vi "filtr2.vi"(8 "threshold":i32=1, 11 "input array":dbl[][](array[numeric])) -> (3 "output array":dbl[][](array[numeric]))   [LabVIEW 2015]
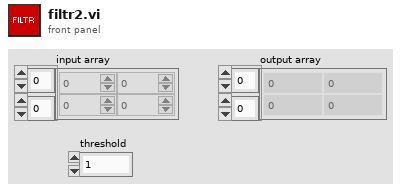
[diagram p1: front panel]
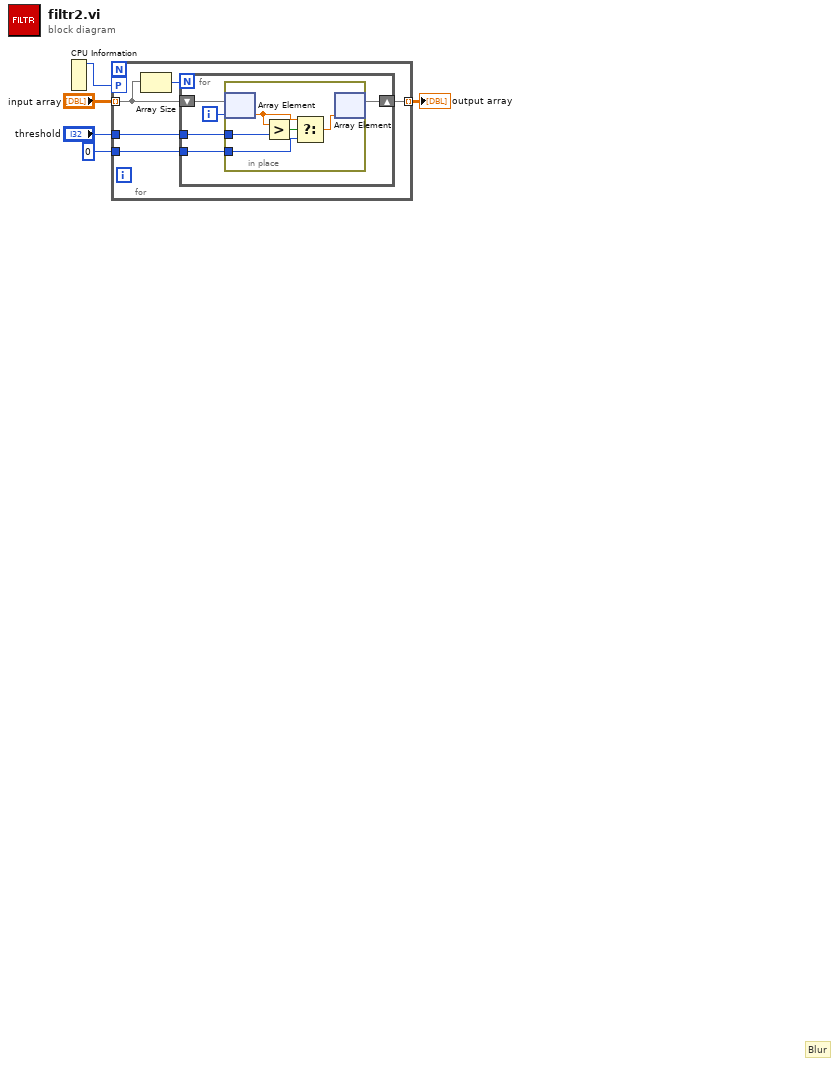
[diagram p0: block diagram]
diagram:
  # "Blur"
  n1 = CPU Information() -> (4:w5:i32)  [unwired: 3 out]
  n2 = for {
    workers-P: w5 -> [_]
    tunnel: "input array" -> [w9] mode=indexing
    tunnel: "threshold" -> [w8]
    tunnel: 0 -> [w7]
    tunnel: [w6] -> w1 mode=indexing
    n3 = Array Size(array=w9) -> (size(s)=w10:i32)
    n4 = for {
      N: w10 -> [_]
      shift-right: [w14] -> w6
      shift-left: w9 -> [w15]
      tunnel: w8 -> [w12]
      tunnel: w7 -> [w11]
      i -> [w13]
      n5 = in-place {
        in-place-border: w12 -> [w19]
        in-place-border: w11 -> [w17]
        n6 = in-place-array #1(w15, w13) -> (w18:dbl)
        n7 = Greater?(x=w18, y=w19) -> (0:w20:bool)
        n8 = Select(t=w18, s=w20, f=w17) -> (s? t:f=w16:dbl)
        n9 = in-place-array #1(w16) -> (w14:dbl[])  [unwired: 1 out]
      }
    }
  }
  "output array" <- w1
